vi "Add Status Channel Tree.vi"(8 "error in (no error)":errorcluster, 11 "Parent Ref in":T1 format="%.0x") -> (0 "error out":errorcluster, 3 "Parent Ref out":T1 format="%.0x")   [LabVIEW 2020, in "Vires VTD System Explorer.lvlib"]
uses:
  Vires VTD System Explorer.lvlib
  <vilib>/NI VeriStand/Custom Device API/Custom Device Item Ref.ctl
  <vilib>/NI VeriStand/Custom Device API/Custom Device Channel.ctl
  <vilib>/NI VeriStand/Custom Device API/Custom Device Channel Type.ctl
  Shared/Constants.vi
  Shared/Vires VTD Shared.lvlib
  <vilib>/NI VeriStand/Custom Device API/Custom Device API.lvlib
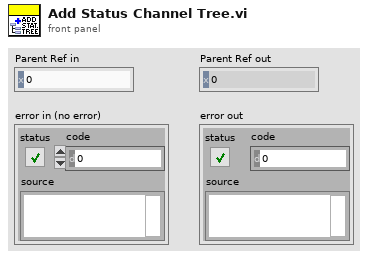
[diagram p1: front panel]
types:
  T1 = typedef "Custom Device API.lvlib/Custom Device Item Ref.ctl" = u64
  T2 = typedef "Custom Device API.lvlib/Custom Device Channel.ctl" = cluster{"Type":T3, "Units":string, "Default Value":dbl, "Faultable":bool, "Scalable":bool}
  T3 = typedef "Custom Device API.lvlib/Custom Device Channel Type.ctl" = enum16{"Input", "Output"}
  T4 = cluster{"Name":string, "Description":string, "Channel":T2}[]
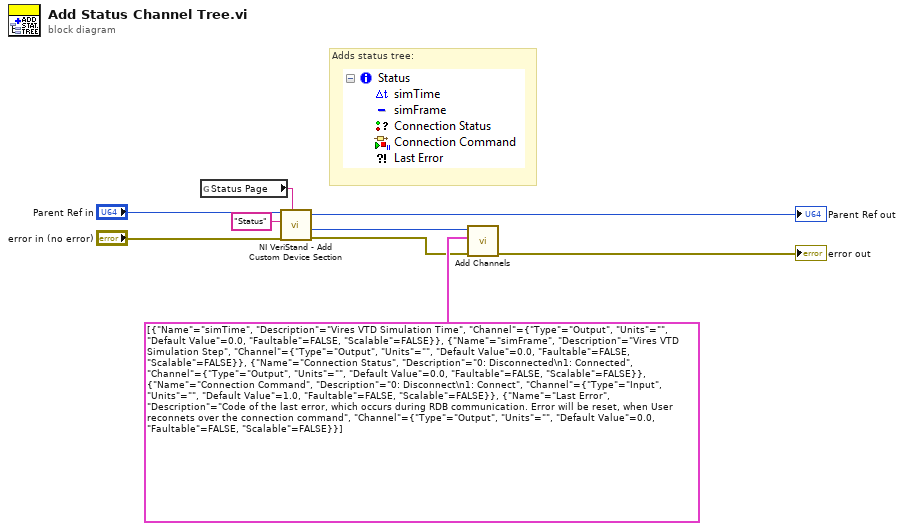
[diagram p0: block diagram]
diagram:
  # "Adds status tree:"
  n1 = global read "Constants.vi" "Status Page"() -> (w3:string)
  n2 = call <vilib>:"NI VeriStand - Add Custom Device Section.vi"("GUID (Default Section)"=w3, "error in (no error)"="error in (no error)", "Section Name"="Status", "Parent Ref in"="Parent Ref in") -> ("error out"=w2:errorcluster, "Section Ptr"=w8:T1, "Parent Ref out"=→"Parent Ref out":T1)  [unwired: 4 in, 1 out]
  n3 = call "Add Channels.vi"("error in (no error)"=w2, "Channels Setup"=T4 [{"Name"="simTime", "Description"="Vires VTD Simulation Time", "Channel"={"Type"=enum."Output", "Units"="", "Default Value"=0.0, "Faultable"=FALSE, "Scalable"=FALSE}}, {"Name"="simFrame", "Description"="Vires VTD Simulation Step", "Channel"={"Type"=enum."Output", "Units"="", "Default Value"=0.0, "Faultable"=FALSE, "Scalable"=FALSE}}, {"Name"="Connection Status", "Description"="0: Disconnected\n1: Connected", "Channel"={"Type"=enum."Output", "Units"="", "Default Value"=0.0, "Faultable"=FALSE, "Scalable"=FALSE}}, {"Name"="Connection Command", "Description"="0: Disconnect\n1: Connect", "Channel"={"Type"=enum."Input", "Units"="", "Default Value"=1.0, "Faultable"=FALSE, "Scalable"=FALSE}}, {"Name"="Last Error", "Description"="Code of the last error, which occurs during RDB communication. Error will be reset, when User reconnets over the connection command", "Channel"={"Type"=enum."Output", "Units"="", "Default Value"=0.0, "Faultable"=FALSE, "Scalable"=FALSE}}], "Section Ptr In"=w8) -> ("error out"=→"error out":errorcluster)  [unwired: 7 in, 1 out]
